vi "Server3.vi"() -> ()   [LabVIEW 2015]
panel:
  out "Message Length":i32
  out "Wavelength data":dbl[][](array[numeric])
  in  "Transmission control":bool
  in  "Sampling Frequency (Hz)":dbl format="%#_13g"
  out "Wavelength Data":string="Wavelength Data"
  in  "Wavelength Data":string="Wavelength Data"
  out "Error out":errorcluster
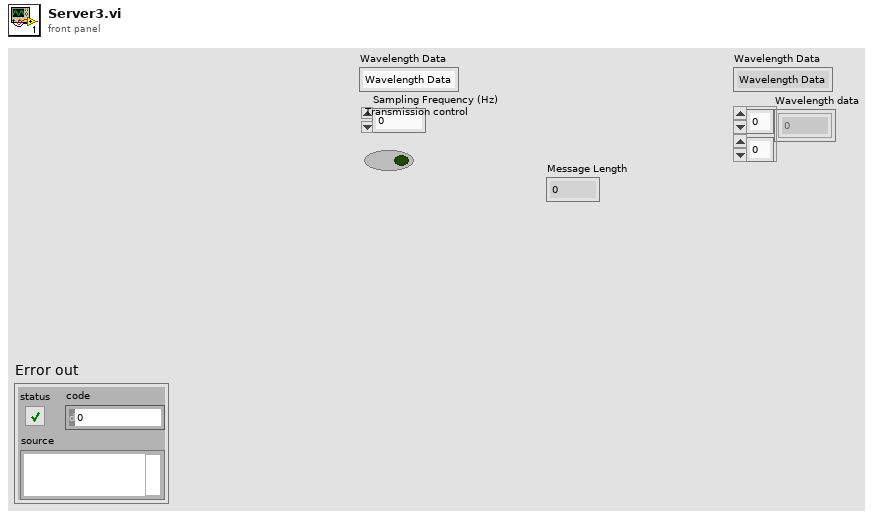
[diagram p1: front panel]
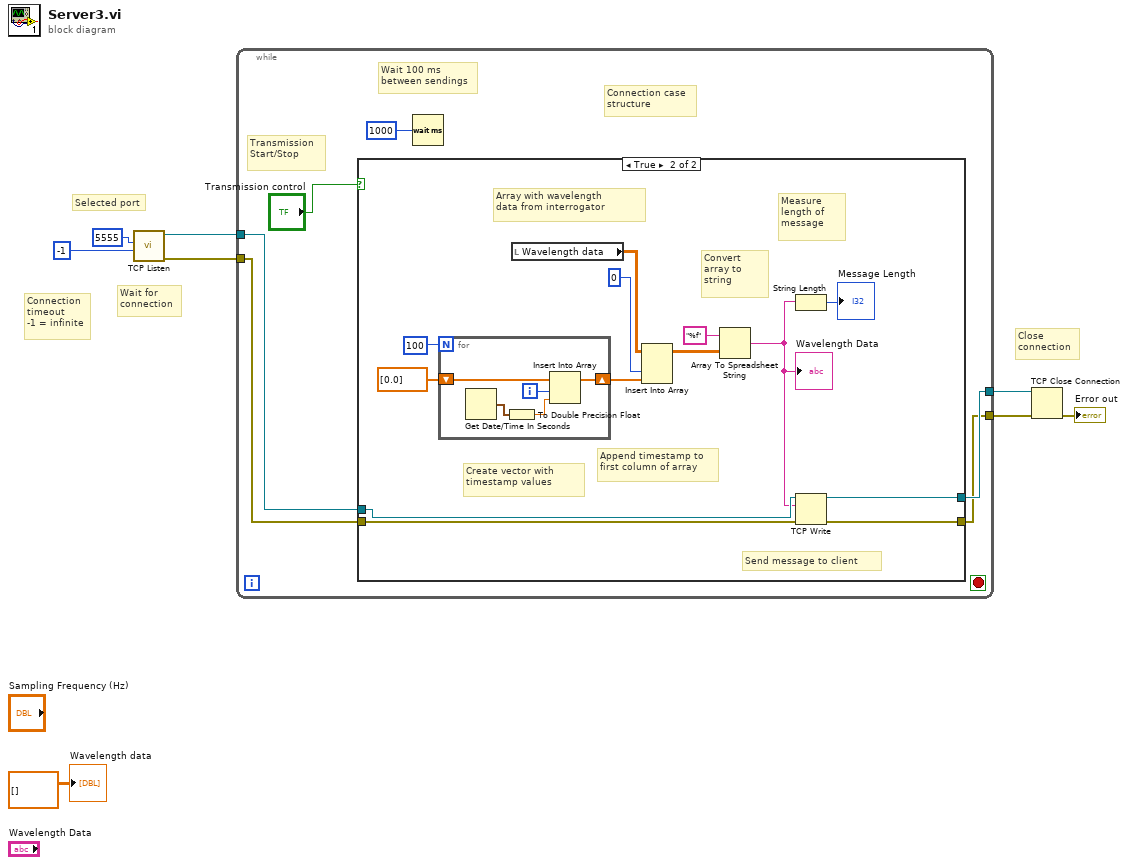
[diagram p0: block diagram]
diagram:
  # "Close \nconnection"
  # "Wait for\nconnection"
  # "Connection\ntimeout\n-1 = infinite"
  # "Selected port"
  n1 = call <vilib>:"TCP Listen.vi"("timeout ms (wait forever: -1)"=-1 ("Timeout [ms]\n (wait forever: -1)"), "port"=u16 5555 ("Port")) -> ("error out"=w4:errorcluster, "connection ID"=w5:refnum<k5>)  [unwired: 5 in, 3 out]
  n2 = while {
    tunnel: w5 -> [w14]
    tunnel: w4 -> [w13]
    tunnel: [w12] -> w3
    tunnel: [w11] -> w2
    stop <- _ stop-if-true
    # "Connection case\nstructure"
    # "Transmission Start/Stop"
    # "Wait 100 ms \nbetween sendings"
    n3 = case shown="True" "Transmission control" {
      tunnel: w14 -> [_ w27]
      tunnel: w13 -> [_ w26]
      tunnel: [_ w25] -> w12
      tunnel: [_ w24] -> w11
      frame False {
      }
      frame True {
        # "Send message to client"
        # "Measure length of message"
        # "Convert array to string"
        # "Append timestamp to first column of array"
        # "Create vector with timestamp values"
        # "Array with wavelength \ndata from interrogator"
        n4 = for {
          N: 100 -> [_]
          shift-right: [w31] -> w21
          shift-left: dbl[] [0.0] -> [w32]
          i -> [w30]
          n5 = Get Date/Time In Seconds() -> (seconds since 1Jan1904=w29:timestamp)
          n6 = To Double Precision Float(number=w29) -> (double precision float=w28:dbl)
          n7 = Insert Into Array(array=w32, index=w30, new element=w28) -> (w31:dbl[])
        }
        n8 = local read "Wavelength data"() -> (w19:dbl[][])
        n9 = Insert Into Array(array=w19, index (col)=0, new element=w21) -> (w17:dbl[][])  [unwired: 1 in]
        n10 = Array To Spreadsheet String(array=w17, 3:"%f" ("format string")) -> (spreadsheet string=w15:string)  [unwired: 1 in]
        "Wavelength Data" <- w15
        n11 = String Length(string=w15) -> (length=→"Message Length":i32)
        n12 = TCP Write(connection ID=w27, data in=w15, error in (no error)=w26) -> (connection ID out=w25:refnum<k5>, error out=w24:errorcluster)  [unwired: 1 in, 1 out]
      }
    }
    n13 = Wait (ms)(milliseconds to wait=u32 1000 ("Wait [ms]")) -> ()  [unwired: 1 out]
  }
  n14 = TCP Close Connection(connection ID=w3, error in (no error)=w2) -> (error out=→"Error out":errorcluster)  [unwired: 1 in, 1 out]
  "Wavelength data" <- dbl[][] []
